vi "Read Typedef Path.vi"(11 "Enum Writer in":refnum<class "Enum Writer.lvclass">) -> (2 "Typedef Path":path, 3 "Enum Writer out":refnum<class "Enum Writer.lvclass">)   [LabVIEW 2013, in "Enum Writer.lvclass"]
doc: "Copyright (c) 2016 Sze Howe Koh\n\nThis Source Code Form is subject to the terms of the Mozilla Public License, v. 2.0. If a copy of the MPL was not distributed with this file, You can obtain one at http://mozilla.org/MPL/2.0/."
uses:
  Enum Writer.lvclass
  Enum Writer.lvclass/Enum Writer.ctl
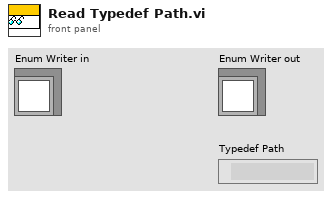
[diagram p1: front panel]
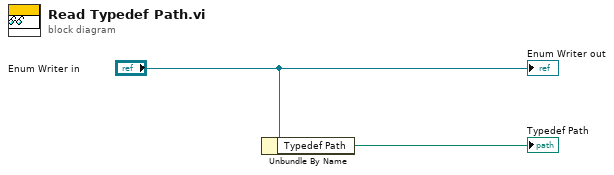
[diagram p0: block diagram]
diagram:
  n1 = Unbundle By Name("Enum Writer in") -> ("Typedef Path"=→"Typedef Path":path)
  "Enum Writer out" <- "Enum Writer in"
